vi "CRYAuto Create Recalled Results.vi"(8 "all or last":i32, 9 "Curve Names in":string[](array[string]), 10 "Curves Selected?":bool[](array[boolean]), 11 "Result Array":T1[](array[typedef]) {"Margin" format="%.2f"}) -> (3 "Resut Out":T1[](array[typedef]) {"Margin" format="%.2f"})   [LabVIEW 2013]
uses:
  Typedef Control/CRYResult Cluster.ctl
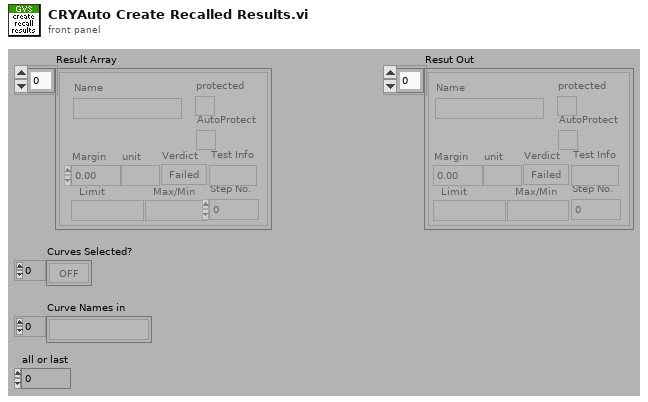
[diagram p1: front panel]
types:
  T1 = typedef "CRYResult Cluster.ctl" = cluster{"Name":string, "Margin":dbl, "unit":string, "Verdict":bool, "Limit":string, "Max/Min":string, "protected":bool, "Step No.":i32, "Test Info":string, "AutoProtect":bool}
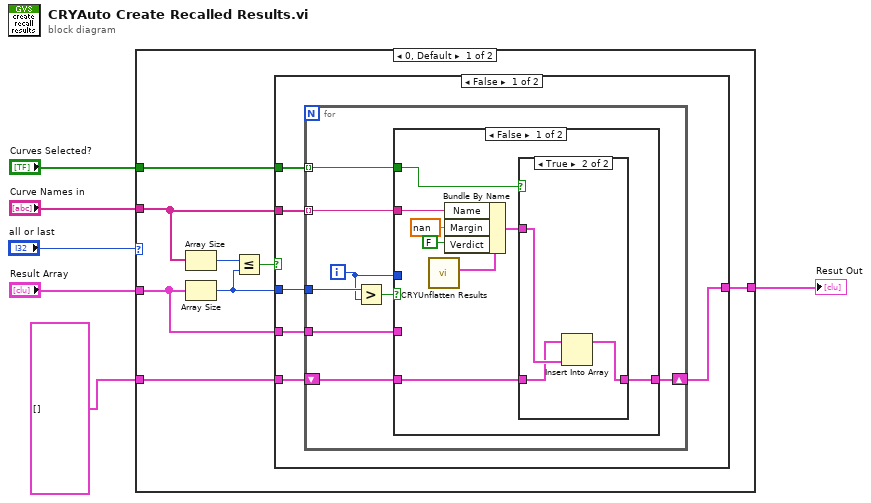
[diagram p0: block diagram]
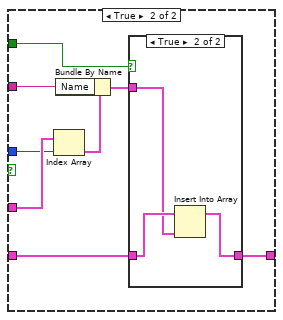
[diagram p3: hidden frame]
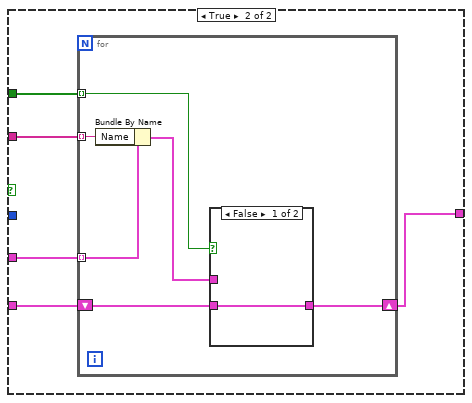
[diagram p5: hidden frame]
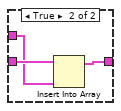
[diagram p6: hidden frame]
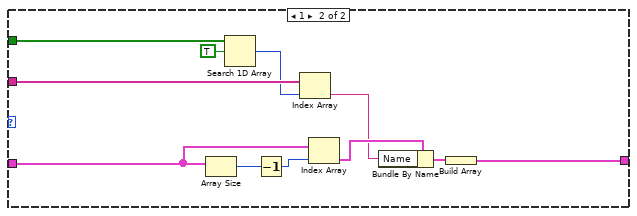
[diagram p7: hidden frame]
diagram:
  n1 = case shown="0, Default" "all or last" {
    tunnel: "Result Array" -> [w11 w73]
    tunnel: "Curve Names in" -> [w9 w76]
    tunnel: "Curves Selected?" -> [w12 w78]
    tunnel: [w8 w68] -> w1
    tunnel: T1[] [] ("appended array") -> [w10 _]
    frame 0, Default {
      n2 = Array Size(array=w9) -> (size(s)=w14:i32)
      n3 = Array Size(array=w11) -> (size(s)=w7:i32)
      n4 = Less Or Equal?(x=w14, y=w7) -> (x <= y?=w13:bool)
      n5 = case shown="False" w13 {
        tunnel: w12 -> [w20 w57]
        tunnel: w11 -> [w17 w56]
        tunnel: w10 -> [w16 w55]
        tunnel: w9 -> [w19 w54]
        tunnel: [w15 w53] -> w8
        tunnel: w7 -> [w18 _]
        frame False {
          n6 = for {
            tunnel: w20 -> [w26] mode=indexing
            tunnel: w19 -> [w23] mode=indexing
            tunnel: w18 -> [w28]
            tunnel: w17 -> [w25]
            shift-right: [w21] -> w15
            shift-left: w16 -> [w22]
            i -> [w24]
            n7 = Greater?(x=w28, y=w24) -> (0:w27:bool)
            n8 = case shown="False" w27 {
              tunnel: w26 -> [w36 w48]
              tunnel: w25 -> [_ w47]
              tunnel: w24 -> [_ w46]
              tunnel: w23 -> [w33 w44]
              tunnel: w22 -> [w35 w42]
              tunnel: [w34 w41] -> w21
              frame False {
                n9 = call "CRYUnflatten Results.vi"() -> ("Result"=w32:T1)  [unwired: 9 in, 2 out]
                n10 = Bundle By Name(cluster=w32, "Name"=w33, "Margin"=nan, "Verdict"=FALSE) -> (w31:T1)
                n11 = case shown="True" w36 {
                  tunnel: w31 -> [_ w40]
                  tunnel: w35 -> [w37 w39]
                  tunnel: [w37 w38] -> w34
                  frame False {
                  }
                  frame True {
                    n12 = Insert Into Array(array=w39, new element=w40) -> (w38:T1[])  [unwired: 1 in]
                  }
                }
              }
              frame True {
                n13 = Index Array(array=w47, index=w46) -> (element=w45:T1)
                n14 = Bundle By Name(cluster=w45, "Name"=w44) -> (w43:T1)
                n15 = case shown="True" w48 {
                  tunnel: w43 -> [_ w51]
                  tunnel: w42 -> [w49 w52]
                  tunnel: [w49 w50] -> w41
                  frame False {
                  }
                  frame True {
                    n16 = Insert Into Array(array=w52, new element=w51) -> (w50:T1[])  [unwired: 1 in]
                  }
                }
              }
            }
          }
        }
        frame True {
          n17 = for {
            tunnel: w57 -> [w63] mode=indexing
            tunnel: w56 -> [w59] mode=indexing
            shift-right: [w61] -> w53
            shift-left: w55 -> [w62]
            tunnel: w54 -> [w60] mode=indexing
            n18 = Bundle By Name(cluster=w59, "Name"=w60) -> (w58:T1)
            n19 = case shown="False" w63 {
              tunnel: w58 -> [_ w66]
              tunnel: w62 -> [w64 w67]
              tunnel: [w64 w65] -> w61
              frame False {
              }
              frame True {
                n20 = Insert Into Array(array=w67, new element=w66) -> (w65:T1[])  [unwired: 1 in]
              }
            }
          }
        }
      }
    }
    frame 1 {
      n21 = Array Size(array=w73) -> (size(s)=w74:i32)
      n22 = Search 1D Array(1D array=w78, element=TRUE) -> (index of element=w75:i32)  [unwired: 1 in]
      n23 = Decrement(x=w74) -> (x-1=w72:i32)
      n24 = Index Array(array=w76, index=w75) -> (element=w70:string)
      n25 = Index Array(array=w73, index=w72) -> (element=w71:T1)
      n26 = Bundle By Name(cluster=w71, "Name"=w70) -> (w69:T1)
      n27 = Build Array(w69) -> (w68:T1[])
    }
  }
  "Resut Out" <- w1
